vi "Write Cooler Enqueuer.vi"(10 "冷却器待入队列":refnum<class "Message Enqueuer.lvclass">, 11 "冷却器的控制器输入":refnum<class "Cooler Controller.lvclass">) -> (3 "冷却器的控制器输出":refnum<class "Cooler Controller.lvclass">)   [LabVIEW 2015, in "Cooler Controller.lvlib" / "Cooler Controller.lvclass"]
doc: "该VI通知控制器当前负责控制的冷却器。如将输入设置为“非法引用句柄”待入队列，则表示控制器当前不对任何冷却器进行控制。"
uses:
  Cooler Controller.lvclass
  <vilib>/ActorFramework/Message Enqueuer/Message Enqueuer.lvclass
  Cooler Controller.lvclass/Cooler Controller.ctl
  Level Controller/Level Controller/Deadband.ctl
  Level Controller/Write Deadband Msg/Write Deadband Msg.lvclass/Write Deadband Msg.ctl
  <vilib>/ActorFramework/Message Enqueuer/Message Enqueuer.lvclass/Message Enqueuer.ctl
  <vilib>/ActorFramework/Message Enqueuer/Enqueue.vi
  <vilib>/ActorFramework/Message Priority Queue/Priority Enqueue.vi
  Level Controller/Write Deadband Msg/Write Deadband Msg.lvclass
  Level Controller/Level Controller/Level Controller.lvclass
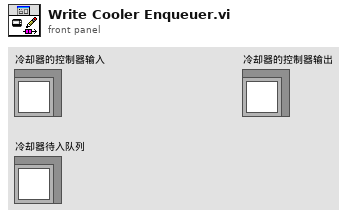
[diagram p1: front panel]
types:
  T1 = typedef "Level Controller.lvlib/Level Controller.lvclass/Deadband.ctl" = cluster{"低":dbl, "高":dbl}
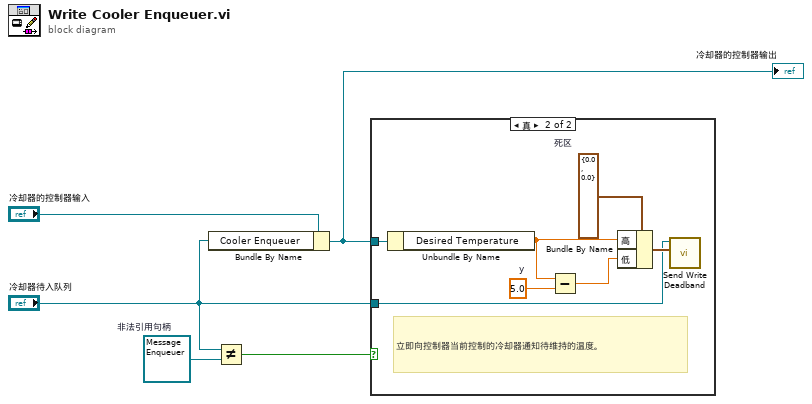
[diagram p0: block diagram]
diagram:
  w4 = refnum<class "Message Enqueuer.lvclass"> refnum  # 非法引用句柄
  n1 = Bundle By Name(cluster="冷却器的控制器输入", "Cooler Enqueuer"="冷却器待入队列") -> (w2:refnum<class "Cooler Controller.lvclass">)
  "冷却器的控制器输出" <- w2
  n2 = Not Equal?(x="冷却器待入队列", y=w4) -> (x != y?=w3:bool)
  n3 = case shown="真" w3 {
    tunnel: w2 -> [_ w12]
    tunnel: "冷却器待入队列" -> [_ w6]
    frame False {
    }
    frame True {
      w10 = 5.0  # y
      w11 = T1 {"低"=0.0, "高"=0.0}  # 死区
      # "立即向控制器当前控制的冷却器通知待维持的温度。"
      n4 = Unbundle By Name(w12) -> ("Desired Temperature"=w9:dbl)
      n5 = Subtract(x=w9, y=w10) -> (x-y=w8:dbl)
      n6 = Bundle By Name(cluster=w11, "高"=w9, "低"=w8) -> (w7:T1)
      n7 = call "Send Write Deadband.vi"("死区"=w7, "消息待入队列"=w6) -> ()  [unwired: 9 in, 1 out]
    }
  }
